vi "check_if_should_flash (SubVI).vi"(0 "Path":path, 3 "Stop below threshold":bool, 4 "Stop threshold":dbl, 5 "Flash lamp?":bool, 6 "Number of cyles\nbetween flashes":i32, 7 "Loop iteration":i32) -> (1 "Should flash":bool, 2 "Curr threshold":dbl)   [LabVIEW 2018]
uses:
  <vilib>/Utility/file.llb/Read From Spreadsheet File (DBL).vi
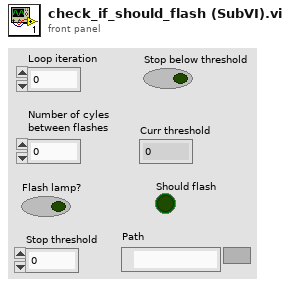
[diagram p1: front panel]
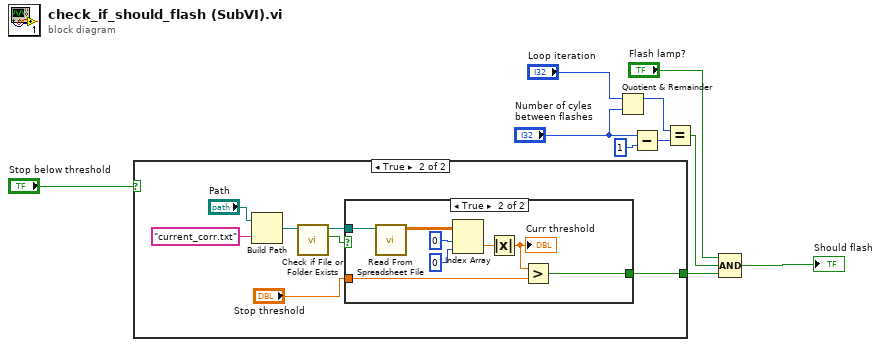
[diagram p0: block diagram]
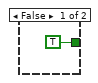
[diagram p2: hidden frame]
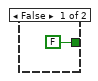
[diagram p3: hidden frame]
diagram:
  n1 = case shown="True" "Stop below threshold" {
    tunnel: [TRUE w17] -> w2
    frame False {
    }
    frame True {
      n2 = Build Path(base path="Path", name or relative path="current_corr.txt") -> (appended path=w16:path)
      n3 = call <vilib>:"Check if File or Folder Exists.vi"("path"=w16) -> ("file or folder exists?"=w15:bool, "dup path"=w14:path)  [unwired: 8 in, 1 out]
      n4 = case shown="True" w15 {
        tunnel: [FALSE w24] -> w17
        tunnel: "Stop threshold" -> [_ w21]
        tunnel: w14 -> [_ w20]
        frame False {
        }
        frame True {
          n5 = call-poly <vilib>:"Read From Spreadsheet File.vi"("file path (dialog if empty)"=w20) -> ("all rows"=w27:dbl[][])  [unwired: 6 in, 4 out]
          n6 = Index Array(array=w27, index (row)=0, index (col)=0 ("disabled index (col)")) -> (element=w23:dbl)
          n7 = Absolute Value(x=w23) -> (abs(x)=w22:dbl)
          "Curr threshold" <- w22
          n8 = Greater?(x=w22, y=w21) -> (0:w24:bool)
        }
      }
    }
  }
  n9 = Quotient & Remainder(x="Loop iteration", y="Number of cyles\nbetween flashes") -> (x-y*floor(x/y)=w7:i32)  [unwired: 1 out]
  n10 = Subtract(x="Number of cyles\nbetween flashes", y=1) -> (x-y=w10:i32)
  n11 = Equal?(x=w7, y=w10) -> (x = y?=w3:bool)
  n12 = Compound Arithmetic op=AND("Flash lamp?", w3, w2) -> (→"Should flash":bool)
